vi "Maintain Inventory.vi"() -> ()   [LabVIEW 2013]
uses:
  Controls/Display Component Line.ctl
  Controls/Components.ctl
  Controls/Component Sub Type.ctl
  Controls/Add Button.ctl
  Controls/Subtract Button.ctl
panel:
  in  "Revert":bool
  in  "Save":bool
  in  "Inventory":T1[](array[typedef])
  # "Maintain Home Lab. Inventory"
  # "Part Number"
  # "Code / Value"
  # "Component Type"
  # "Sub Type"
  # "Quantity"
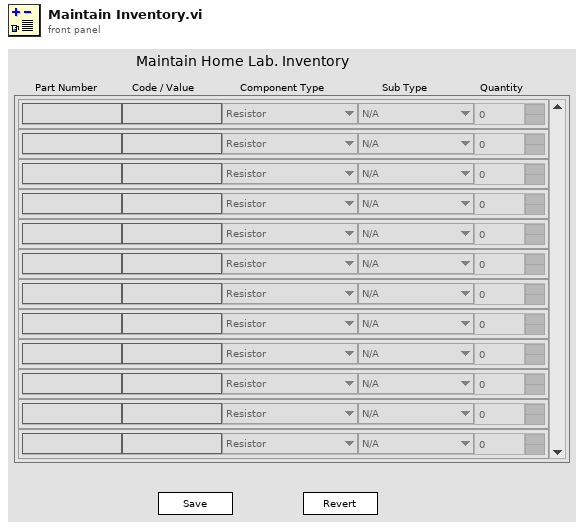
[diagram p1: front panel]
types:
  T1 = typedef "Display Component Line.ctl" = cluster{"Part Number":string, "Code (Value)":string, "Component Type":T2, "Component Subtype":T3, "Quantity":u32, "Add":T4, "Subtract":T5}
  T2 = typedef "Components.ctl" = enum16{"Resistor", "Capacitor", "Diode", "Voltage Regulator"}
  T3 = typedef "Component Sub Type.ctl" = enum16{"N/A", "Ceramic", "Electrolitic", "Zenner", "NPN", "PNP"}
  T4 = typedef "Add Button.ctl" = bool
  T5 = typedef "Subtract Button.ctl" = bool
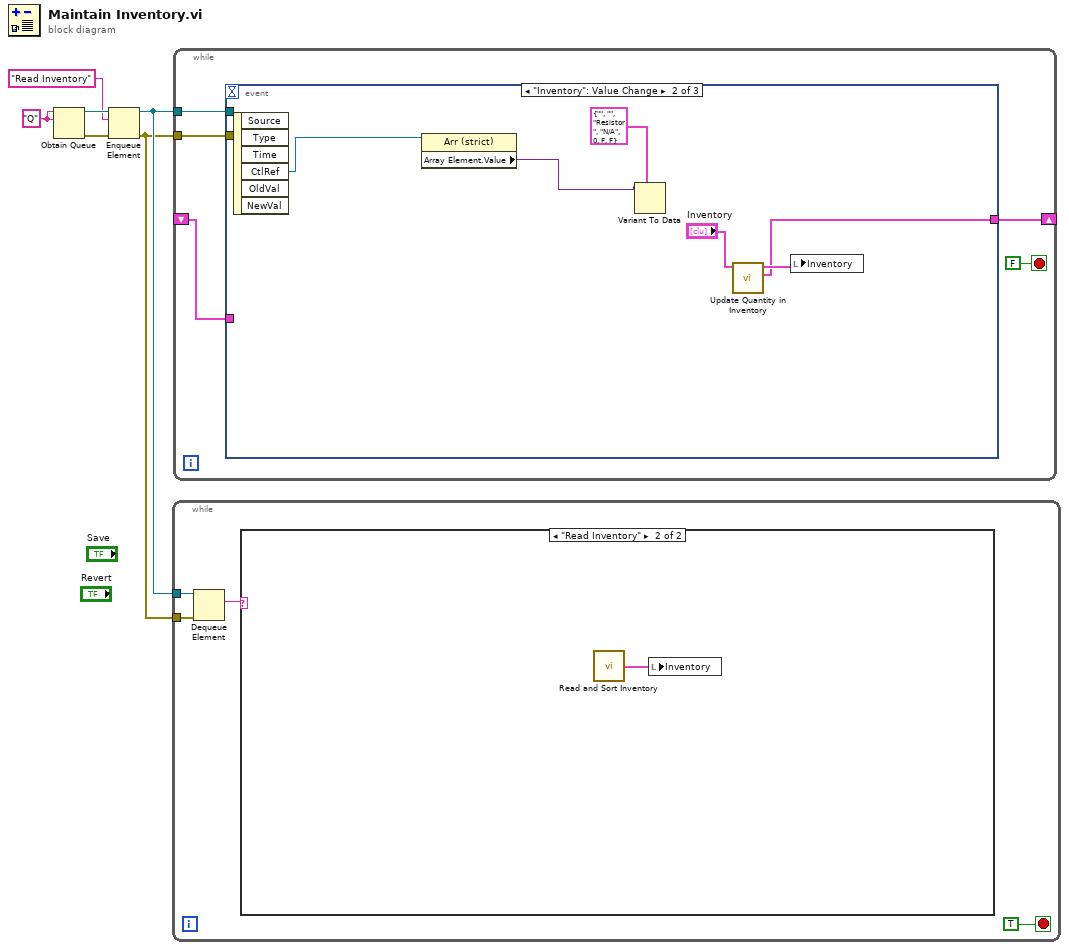
[diagram p0: block diagram]
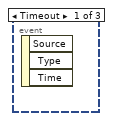
[diagram p3: hidden frame]
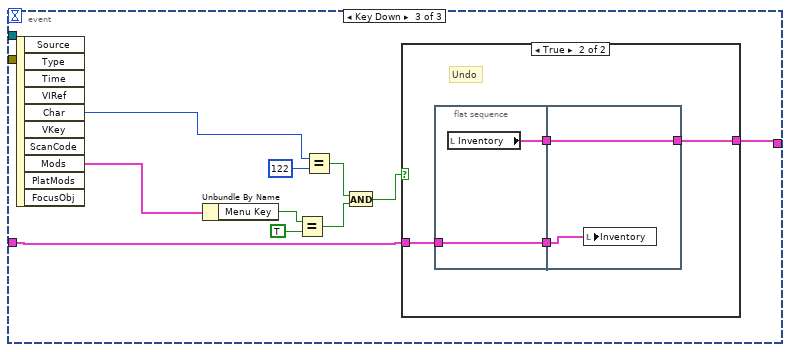
[diagram p4: hidden frame]
diagram:
  w6 = "Q"
  n1 = Obtain Queue(name (unnamed)=w6, element data type=w6) -> (queue out=w4:refnum<queue>, error out=w5:errorcluster)  [unwired: 3 in, 1 out]
  n2 = Enqueue Element(queue=w4, element="Read Inventory", error in (no error)=w5) -> (queue out=w2:refnum<queue>, error out=w1:errorcluster)  [unwired: 1 in, 1 out]
  n3 = while {
    tunnel: w2 -> [w9]
    tunnel: w1 -> [w10]
    stop <- TRUE stop-if-true
    n4 = Dequeue Element(queue=w9, error in (no error)=w10) -> (element=w8:string)  [unwired: 1 in, 3 out]
    n5 = case shown="\"Read Inventory\"" w8 {
      frame Default {
      }
      frame "Read Inventory" {
        n6 = call "Read and Sort Inventory.vi"() -> ("Array"=w11:T1[])  [unwired: 1 in]
        n7 = local write "Inventory"(w11) -> ()
      }
    }
  }
  n8 = while {
    tunnel: w2 -> [w15]
    tunnel: w1 -> [w14]
    shift-right: [w13] -> _
    shift-left: _ -> [w12]
    stop <- FALSE stop-if-true
    n9 = event shown="[1] \"Inventory\": Value Change" {
      selector: _ -> [_ _ _]
      dyn-events: _ -> [_ _ _]
      timeout: _ -> [_ _ _]
      tunnel: w15 -> [_ _ _]
      tunnel: w14 -> [_ _ _]
      tunnel: [_ w17 w23] -> w13
      tunnel: w12 -> [_ _ w24]
      event Timeout {
        n10 = event-data() -> ()  [unwired: 1 in, 3 out]
      }
      event "Inventory": Value Change {
        n11 = event-data() -> ("CtlRef"=w20:refnum<vi>)  [unwired: 1 in, 5 out]
        n12 = property class="Arr (strict)"(reference=w20) -> ("Array Element.Value"=w22:variant)  [unwired: 1 in, 2 out]
        n13 = Variant To Data(type=T1 {"Part Number"="", "Code (Value)"="", "Component Type"=enum."Resistor", "Component Subtype"=enum."N/A", "Quantity"=0, "Add"=FALSE, "Subtract"=FALSE} ("Display Components Line"), Variant=w22) -> ()  [unwired: 1 in, 2 out]
        n14 = call "Update Quantity in Inventory.vi"("Inventory In"="Inventory") -> ("Inventory Out  for Undu2"=w17:T1[], "Inventory Out"=w19:T1[])  [unwired: 8 in, 1 out]
        n15 = local write "Inventory"(w19) -> ()
      }
      event Key Down {
        n16 = event-data() -> ("Char"=w29:i16, "Mods"=w32:cluster{"Num Pad":bool, "Menu Key":bool})  [unwired: 1 in, 8 out]
        n17 = Unbundle By Name(w32) -> ("Menu Key"=w31:bool)
        n18 = Equal?(x=w31, y=TRUE) -> (x = y?=w26:bool)
        n19 = Equal?(x=w29, y=i16 122) -> (x = y?=w27:bool)
        n20 = And(x=w27, y=w26) -> (x .and. y?=w25:bool)
        n21 = case shown="True" w25 {
          tunnel: w24 -> [w33 w34]
          tunnel: [w33 w36] -> w23
          frame False {
          }
          frame True {
            # "Undo"
            n22 = flat-sequence {
              tunnel: [w39] -> w37
              tunnel: [w38] -> w35
              tunnel: w34 -> [w38]
              tunnel: [w41] -> w36
              tunnel: w37 -> [w41]
              tunnel: w35 -> [w40]
              frame #0 {
                n23 = local read "Inventory"() -> (w39:T1[])
              }
              frame #1 {
                n24 = local write "Inventory"(w40) -> ()
              }
            }
          }
        }
      }
    }
  }
